vi "System Performace Tests.vi"() -> ()   [LabVIEW 2021]
uses:
  Source/Support/Nodes/abs_Node/Status.ctl
  Source/System/Support/Stop Status Type.ctl
  Source/System/bt_System.lvclass
  Source/Support/Nodes/Decorators/Repeater/Support/Finish On - Type.ctl
  Source/System/bt_System.lvclass/bt_System.ctl
  Source/System/Properties/Write Behaviour Tree.vi
  Source/BT.lvlib
  Source/Support/Nodes/Decorators/Repeater/bt_Repeater.lvclass
  Source/Support/Nodes/abs_Node/bt_Node.lvclass
panel:
  out "Status":T1
  out "Timeout?":bool
  out "x/y":dbl format="%#_6p"
  out "Status 2":T2
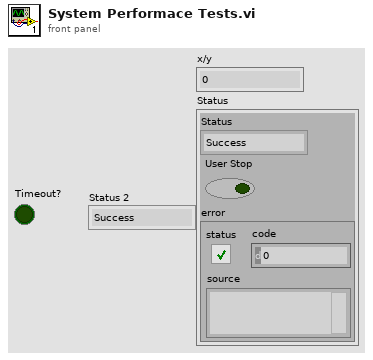
[diagram p1: front panel]
types:
  T1 = typedef "BT.lvlib/bt_System.lvclass/Stop Status Type.ctl" = cluster{"Status":T2, "User Stop":bool, "error":errorcluster}
  T2 = typedef "BT.lvlib/bt_Node.lvclass/Status.ctl" = enum16{"Success", "Failure", "Running"}
  T3 = typedef "BT.lvlib/bt_Repeater.lvclass/Finish On - Type.ctl" = enum16{"Success", "Failure", "Never"}
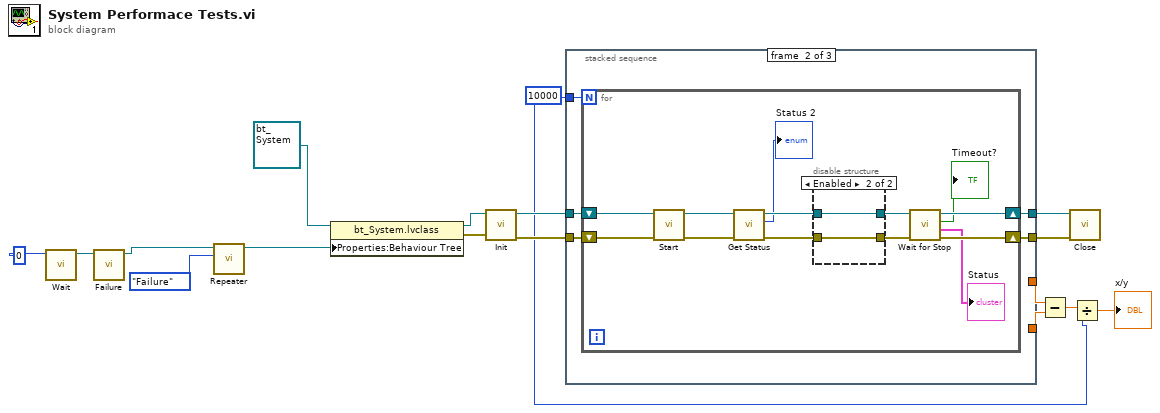
[diagram p0: block diagram]
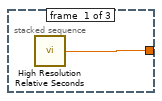
[diagram p2: hidden frame]
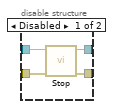
[diagram p3: hidden frame]
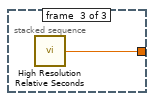
[diagram p4: hidden frame]
diagram:
  w4 = 10000
  n1 = call "Wait.vi"("Time (ms)"=u32 0) -> ("Node Out"=w2:refnum<class "bt_Node.lvclass">)  [unwired: 10 in]
  n2 = call "Failure.vi"("Node In"=w2) -> ("Node"=w1:refnum<class "bt_Node.lvclass">)  [unwired: 10 in]
  n3 = call "Repeater.vi"("Finish On"=Finish_On_-_Type."Failure", "Node In"=w1) -> ("Node Out"=w10:refnum<class "bt_Node.lvclass">)  [unwired: 9 in]
  n4 = property class="bt_System.lvclass"(reference=refnum<class "bt_System.lvclass"> refnum ("bt_System in"), "Properties:Behaviour Tree"=w10) -> (reference out=w11:refnum<class "bt_System.lvclass">, error out=w13:errorcluster)  [unwired: 1 in]
  n5 = call "Init.vi"("error in (no error)"=w13, "bt_System in"=w11) -> ("error out"=w16:errorcluster, "bt_System out"=w17:refnum<class "bt_System.lvclass">)  [unwired: 8 in]
  n6 = stacked-sequence {
    tunnel: w17 -> [_ w23 _]
    tunnel: w16 -> [_ w22 _]
    tunnel: [_ w21 _] -> w15
    tunnel: [_ w20 _] -> w14
    tunnel: [w18 _ _] -> w6
    tunnel: [_ _ w43] -> w7
    tunnel: w4 -> [_ w19 _]
    frame #0 {
      n7 = call <vilib>:"High Resolution Relative Seconds.vi"() -> ("relative seconds"=w18:dbl)
    }
    frame #1 {
      n8 = for {
        N: w19 -> [_]
        shift-right: [w27] -> w21
        shift-left: w23 -> [w36]
        shift-right: [w25] -> w20
        shift-left: w22 -> [w35]
        n9 = call "Start.vi"("error in (no error)"=w35, "bt_System in"=w36) -> ("error out"=w34:errorcluster, "bt_System out"=w33:refnum<class "bt_System.lvclass">)  [unwired: 8 in]
        n10 = call "Get Status.vi"("error in (no error)"=w34, "bt_System in"=w33) -> ("error out"=w31:errorcluster, "Status"=→"Status 2":T2, "bt_System out"=w32:refnum<class "bt_System.lvclass">)  [unwired: 7 in]
        n11 = disable-structure shown="Enabled" {
          disable-tunnel: w32 -> [w40 w42]
          disable-tunnel: w31 -> [w39 w41]
          disable-tunnel: [w38 w41] -> w29
          disable-tunnel: [w37 w42] -> w28
          frame Disabled {
            n12 = call "Stop.vi"("error in (no error)"=w39, "bt_System in"=w40) -> ("error out"=w38:errorcluster, "bt_System out"=w37:refnum<class "bt_System.lvclass">)  [unwired: 8 in]
          }
          frame Enabled {
          }
        }
        n13 = call "Wait for Stop.vi"("error in (no error)"=w29, "bt_System in"=w28) -> ("error"=w25:errorcluster, "Status"=→"Status":T1, "Timeout?"=→"Timeout?":bool, "bt_System out"=w27:refnum<class "bt_System.lvclass">)  [unwired: 6 in]
      }
    }
    frame #2 {
      n14 = call <vilib>:"High Resolution Relative Seconds.vi"() -> ("relative seconds"=w43:dbl)
    }
  }
  n15 = Subtract(x=w7, y=w6) -> (x-y=w5:dbl)
  n16 = call-dynamic "Close.vi"("error in (no error)"=w14, "bt_System in"=w15) -> ()  [unwired: 8 in, 2 out]
  n17 = Divide(x=w5, y=w4) -> (x/y=→"x/y":dbl)
